vi "Actor Teardown Core.vi"(7 "Actor":refnum<class "Actor.lvclass">, 10 "Error":errorcluster, 11 "Destroying Self Actor State in":refnum<class "Destroying Self Actor State.lvclass">) -> (0 "error out":errorcluster, 2 "Teardown?":bool)   [LabVIEW 2021, in "LVCAM.lvlib" / "Destroying Self Actor State.lvclass"]
uses:
  Destroying Self Actor State.lvclass
  Actor/Actor.lvclass
  Self Actor/Self Actor.lvclass
  Msgs/Actor Last Ack/Actor Last Ack Msg Strategy/Actor Last Ack Msg Strategy.lvclass
  C:/git/LabVIEW-Composed-Actor-Model-LVCAM/LabVIEW-Composed-Actor-Model-LVCAM/LVCAM/LVCAM/Msg Strategy/Msg Strategy.lvclass
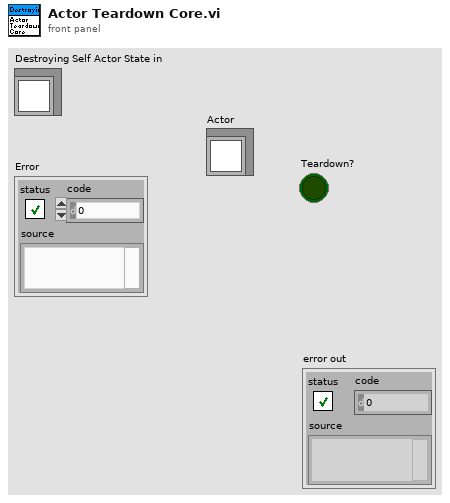
[diagram p1: front panel]
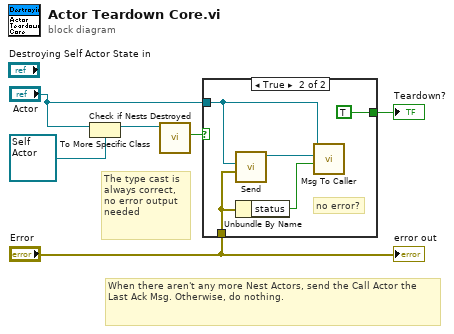
[diagram p0: block diagram]
diagram:
  # "The type cast is always correct, no error output needed"
  # "When there aren't any more Nest Actors, send the Call Actor the Last Ack Msg. Otherwise, do nothing."
  n1 = To More Specific Class(target class=refnum<class "Self Actor.lvclass"> refnum ("LVCAM.lvlib:Self Actor.lvclass"), reference="Actor") -> (specific class reference=w2:refnum<class "Self Actor.lvclass">)  [unwired: 1 in, 1 out]
  n2 = call "Check if Nests Destroyed.vi"("Self Actor"=w2) -> ("Nested Actors Destroyed?"=w5:bool)  [unwired: 10 in]
  n3 = case shown="True" w5 {
    tunnel: "Actor" -> [_ w9]
    tunnel: "Error" -> [_ w10]
    tunnel: [_ TRUE ("Destroyed?")] -> w6
    frame False {
    }
    frame True {
      # "no error?"
      n4 = call "Send.vi"("Nested Error"=w10, "Nested Actor"=w9) -> ("Actor Last Ack Msg Strategy out"=w8:refnum<class "Actor Last Ack Msg Strategy.lvclass">)  [unwired: 9 in]
      n5 = Unbundle By Name(w10) -> ("status"=w7:bool)
      n6 = call-dynamic "Msg To Caller.vi"("Priority Msg?"=w7, "Msg"=w8, "Actor in"=w9) -> ()  [unwired: 8 in, 1 out]
    }
  }
  "Teardown?" <- w6
  "error out" <- "Error"
